vi "Banana.vi"(11 "Boolean":bool) -> (3 "Boolean 2":bool)   [LabVIEW 2020]
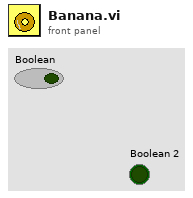
[diagram p1: front panel]
types:
  T1 = typedef "Sound Output Task ID.ctl" = u32
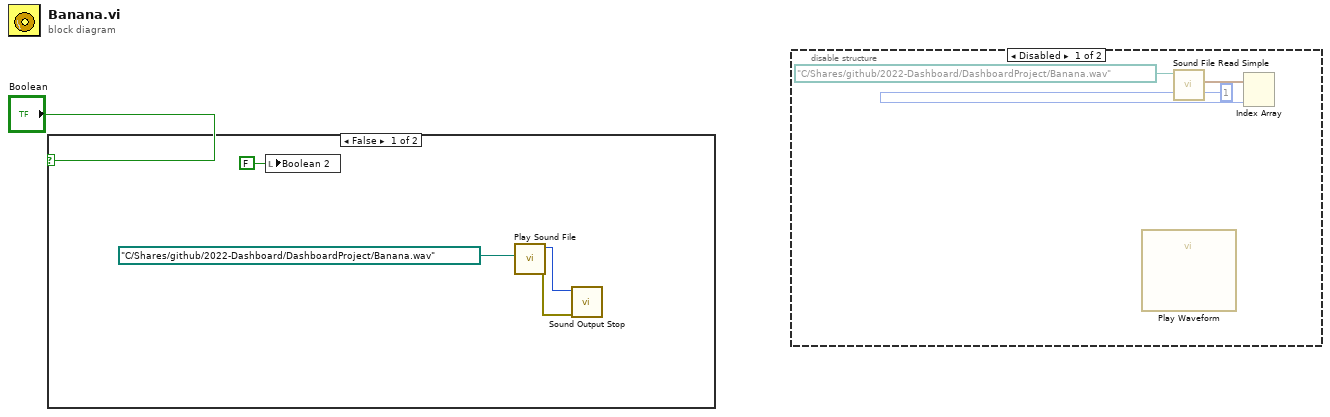
[diagram p0: block diagram]
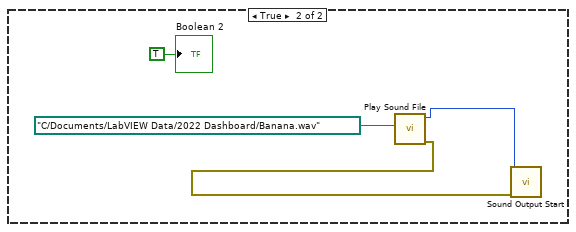
[diagram p3: hidden frame]
diagram:
  n1 = case shown="False" "Boolean" {
    frame False {
      n2 = local write "Boolean 2"(FALSE ("Boolean 2")) -> ()
      n3 = call <vilib>:"Play Sound File.vi"("path"=path "C:/Shares/github/2022-Dashboard/DashboardProject/Banana.wav") -> ("error out"=w2:errorcluster, "task ID"=w3:T1)  [unwired: 9 in]
      n4 = call <vilib>:"Sound Output Stop.vi"("error in (no error)"=w2, "task ID"=w3) -> ()  [unwired: 8 in, 2 out]
    }
    frame True {
      n5 = call <vilib>:"Play Sound File.vi"("path"=path "C:/Documents/LabVIEW Data/2022 Dashboard/Banana.wav") -> ("error out"=w7:errorcluster, "task ID"=w6:T1)  [unwired: 9 in]
      n6 = call <vilib>:"Sound Output Start.vi"("error in (no error)"=w7, "task ID"=w6) -> ()  [unwired: 8 in, 2 out]
      "Boolean 2" <- TRUE ("Boolean 2")
    }
  }
  n7 = disable-structure shown="Disabled" {
    frame Disabled {
      n8 = call "Play Waveform"() -> ("Data"=w13:dynamicdata)  [unwired: 18 in, 1 out]
      n9 = call <vilib>:"Sound File Read Simple.vi"("path"=path "C:/Shares/github/2022-Dashboard/DashboardProject/Banana.wav") -> ("data"=w12:waveform(dbl)[])  [unwired: 7 in, 3 out]
      n10 = Index Array(array=w12, index #2=1 ("index")) -> ()  [unwired: 1 in, 2 out]
    }
    frame Enabled {
    }
  }
